vi "Cluster to String array.vi"(11 "input cluster":T11) -> (3 "appended array":string[][](array[string]))   [LabVIEW 2019, in "HardwareSetup_model001.lvlib" / "HardwareSetup_model001.lvclass"]
uses:
  HardwareSetup_model001.lvclass
  LIN.ctl
  Digital IO.ctl
  DMM.ctl
  Oscilloscope.ctl
  PLC.ctl
  ElectronicLoad.ctl
  PowerSupply.ctl
  CAN.ctl
  Programming.ctl
  Scanner.ctl
  HardwareSetup_model001.lvlib
panel:
  # "LIN_4"
  # "LIN_3"
  # "LIN_2"
  # "LIN_1"
  # "Digital IO_4"
  # "Digital IO_3"
  # "Digital IO_2"
  # "Digital IO_1"
  # "DMM_4"
  # "DMM_3"
  # "DMM_2"
  # "DMM_1"
  # "Oscilloscope_4"
  # "Oscilloscope_3"
  # "Oscilloscope_2"
  # "Oscilloscope_1"
  # "PLC_1"
  # "ElectronicLoad_4"
  # "ElectronicLoad_3"
  # "ElectronicLoad_2"
  # "ElectronicLoad_1"
  # "PowerSupply_4"
  # "PowerSupply_3"
  # "PowerSupply_2"
  # "PowerSupply_1"
  # "CAN_4"
  # "CAN_3"
  # "CAN_2"
  # "CAN_1"
  # "Programming_2"
  # "Programming_1"
  # "Scanner_4"
  # "Scanner_3"
  # "Scanner_2"
  # "Scanner_1"
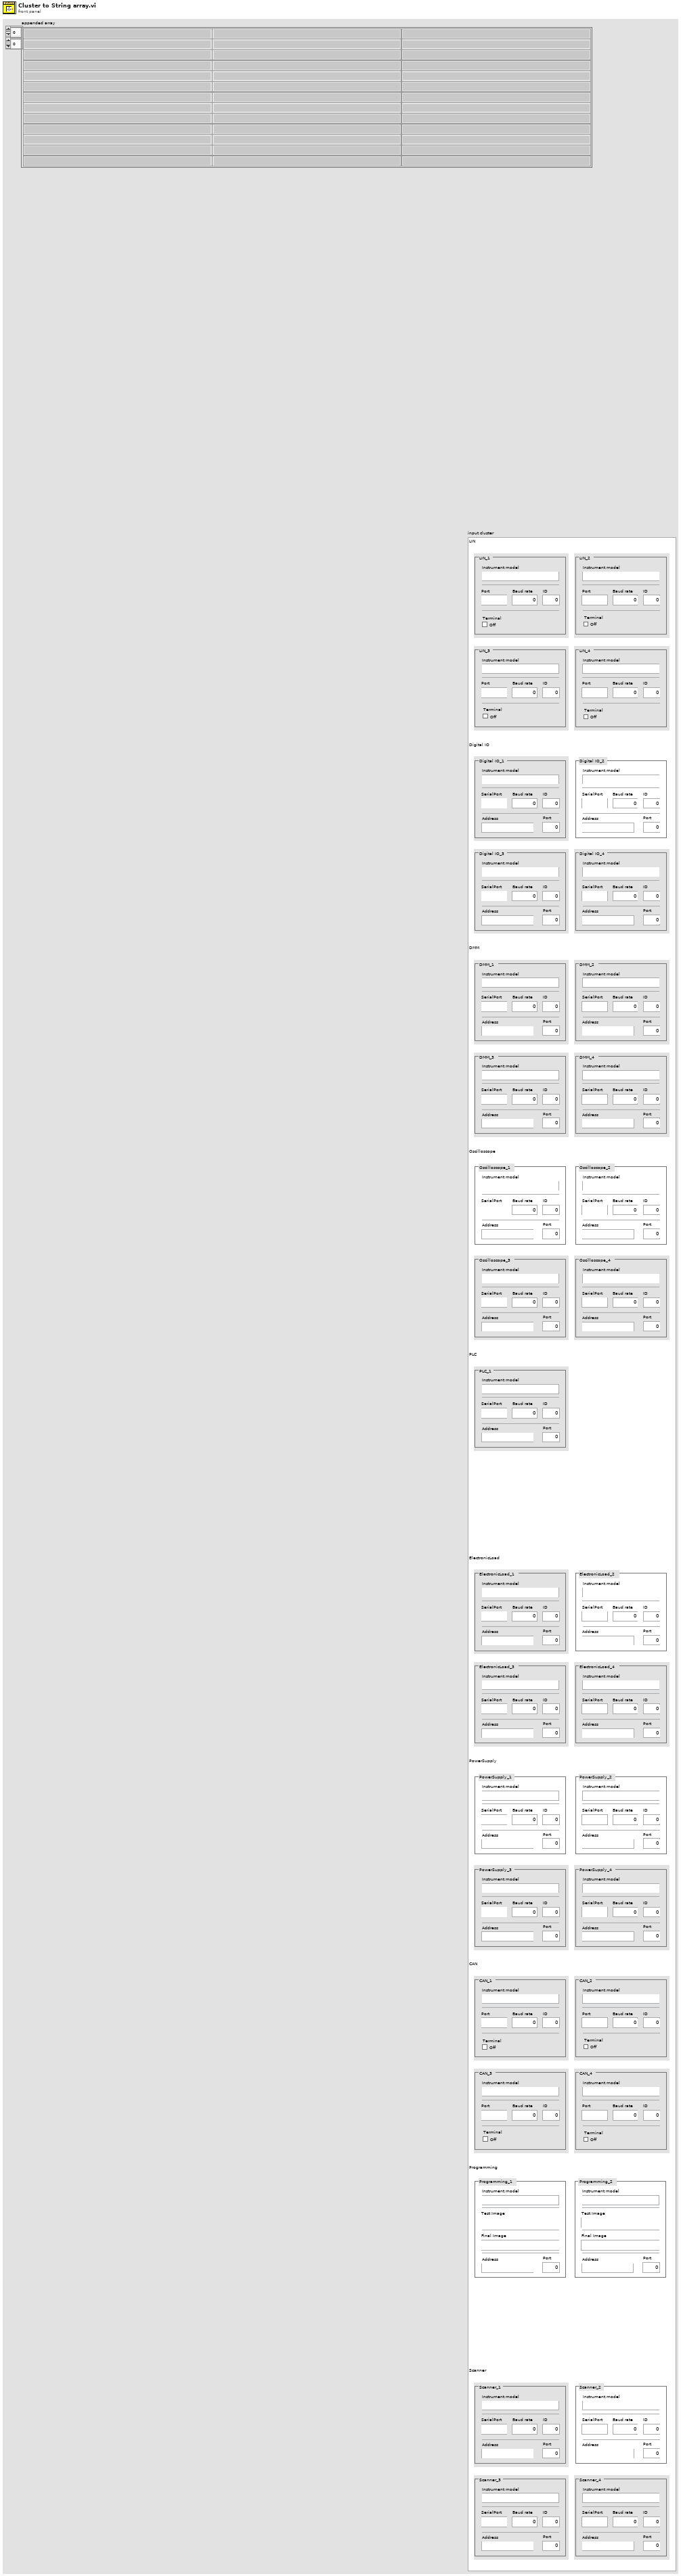
[diagram p1: front panel]
types:
  T1 = typedef "HardwareSetup_model001.lvlib/LIN.ctl" = cluster{"LIN 1":cluster{"Instrument model":string, "Port":string, "Baud rate":i32, "ID":i32, "Terminal":bool}, "LIN 2":cluster{"Instrument model":string, "Port":string, "Baud rate":i32, "ID":i32, "Terminal":bool}, "LIN 3":cluster{"Instrument model":string, "Port":string, "Baud rate":i32, "ID":i32, "Terminal":bool}, "LIN 4":cluster{"Instrument model":string, "Port":string, "Baud rate":i32, "ID":i32, "Terminal":bool}}
  T2 = typedef "HardwareSetup_model001.lvlib/Digital IO.ctl" = cluster{"Digital IO 1":cluster{"SerialPort":string, "Baud rate":i32, "Address":string, "ID":i32, "Port":i32, "Instrument model":string}, "Digital IO 2":cluster{"SerialPort":string, "Baud rate":i32, "Address":string, "ID":i32, "Port":i32, "Instrument model":string}, "Digital IO 3":cluster{"SerialPort":string, "Baud rate":i32, "Address":string, "ID":i32, "Port":i32, "Instrument model":string}, "Digital IO 4":cluster{"SerialPort":string, "Baud rate":i32, "Address":string, "ID":i32, "Port":i32, "Instrument model":string}}
  T3 = typedef "HardwareSetup_model001.lvlib/DMM.ctl" = cluster{"DMM 1":cluster{"SerialPort":string, "Baud rate":i32, "Address":string, "ID":i32, "Port":i32, "Instrument model":string}, "DMM 2":cluster{"SerialPort":string, "Baud rate":i32, "Address":string, "ID":i32, "Port":i32, "Instrument model":string}, "DMM 3":cluster{"SerialPort":string, "Baud rate":i32, "Address":string, "ID":i32, "Port":i32, "Instrument model":string}, "DMM 4":cluster{"SerialPort":string, "Baud rate":i32, "Address":string, "ID":i32, "Port":i32, "Instrument model":string}}
  T4 = typedef "HardwareSetup_model001.lvlib/Oscilloscope.ctl" = cluster{"Oscilloscope 1":cluster{"SerialPort":string, "Baud rate":i32, "Address":string, "ID":i32, "Port":i32, "Instrument model":string}, "Oscilloscope 2":cluster{"SerialPort":string, "Baud rate":i32, "Address":string, "ID":i32, "Port":i32, "Instrument model":string}, "Oscilloscope 3":cluster{"SerialPort":string, "Baud rate":i32, "Address":string, "ID":i32, "Port":i32, "Instrument model":string}, "Oscilloscope 4":cluster{"SerialPort":string, "Baud rate":i32, "Address":string, "ID":i32, "Port":i32, "Instrument model":string}}
  T5 = typedef "HardwareSetup_model001.lvlib/PLC.ctl" = cluster{"PLC 1":cluster{"SerialPort":string, "Baud rate":i32, "Address":string, "ID":i32, "Port":i32, "Instrument model":string}}
  T6 = typedef "HardwareSetup_model001.lvlib/ElectronicLoad.ctl" = cluster{"ElectronicLoad 1":cluster{"SerialPort":string, "Baud rate":i32, "Address":string, "ID":i32, "Port":i32, "Instrument model":string}, "ElectronicLoad 2":cluster{"SerialPort":string, "Baud rate":i32, "Address":string, "ID":i32, "Port":i32, "Instrument model":string}, "ElectronicLoad 3":cluster{"SerialPort":string, "Baud rate":i32, "Address":string, "ID":i32, "Port":i32, "Instrument model":string}, "ElectronicLoad 4":cluster{"SerialPort":string, "Baud rate":i32, "Address":string, "ID":i32, "Port":i32, "Instrument model":string}}
  T7 = typedef "HardwareSetup_model001.lvlib/PowerSupply.ctl" = cluster{"PowerSupply 1":cluster{"SerialPort":string, "Baud rate":i32, "Address":string, "ID":i32, "Port":i32, "Instrument model":string}, "PowerSupply 2":cluster{"SerialPort":string, "Baud rate":i32, "Address":string, "ID":i32, "Port":i32, "Instrument model":string}, "PowerSupply 3":cluster{"SerialPort":string, "Baud rate":i32, "Address":string, "ID":i32, "Port":i32, "Instrument model":string}, "PowerSupply 4":cluster{"SerialPort":string, "Baud rate":i32, "Address":string, "ID":i32, "Port":i32, "Instrument model":string}}
  T8 = typedef "HardwareSetup_model001.lvlib/CAN.ctl" = cluster{"CAN 1":cluster{"Instrument model":string, "Port":string, "Baud rate":i32, "ID":i32, "Terminal":bool}, "CAN 2":cluster{"Instrument model":string, "Port":string, "Baud rate":i32, "ID":i32, "Terminal":bool}, "CAN 3":cluster{"Instrument model":string, "Port":string, "Baud rate":i32, "ID":i32, "Terminal":bool}, "CAN 4":cluster{"Instrument model":string, "Port":string, "Baud rate":i32, "ID":i32, "Terminal":bool}}
  T9 = typedef "HardwareSetup_model001.lvlib/Programming.ctl" = cluster{"Programming 1":cluster{"Test Image":string, "Address":string, "Port":i32, "Instrument model":string, "Final Image":string}, "Programming 2":cluster{"Test Image":string, "Address":string, "Port":i32, "Instrument model":string, "Final Image":string}}
  T10 = typedef "HardwareSetup_model001.lvlib/Scanner.ctl" = cluster{"Scanner 1":cluster{"SerialPort":string, "Baud rate":i32, "Address":string, "ID":i32, "Port":i32, "Instrument model":string}, "Scanner 2":cluster{"SerialPort":string, "Baud rate":i32, "Address":string, "ID":i32, "Port":i32, "Instrument model":string}, "Scanner 3":cluster{"SerialPort":string, "Baud rate":i32, "Address":string, "ID":i32, "Port":i32, "Instrument model":string}, "Scanner 4":cluster{"SerialPort":string, "Baud rate":i32, "Address":string, "ID":i32, "Port":i32, "Instrument model":string}}
  T11 = cluster{"LIN":T1, "Digital IO":T2, "DMM":T3, "Oscilloscope":T4, "PLC":T5, "ElectronicLoad":T6, "PowerSupply":T7, "CAN":T8, "Programming":T9, "Scanner":T10}
  T12 = cluster{"SerialPort":string, "Baud rate":i32, "Address":string, "ID":i32, "Port":i32, "Instrument model":string}[]
  T13 = cluster{"Instrument model":string, "Port":string, "Baud rate":i32, "ID":i32, "Terminal":bool}[]
  T14 = cluster{"Test Image":string, "Address":string, "Port":i32, "Instrument model":string, "Final Image":string}[]
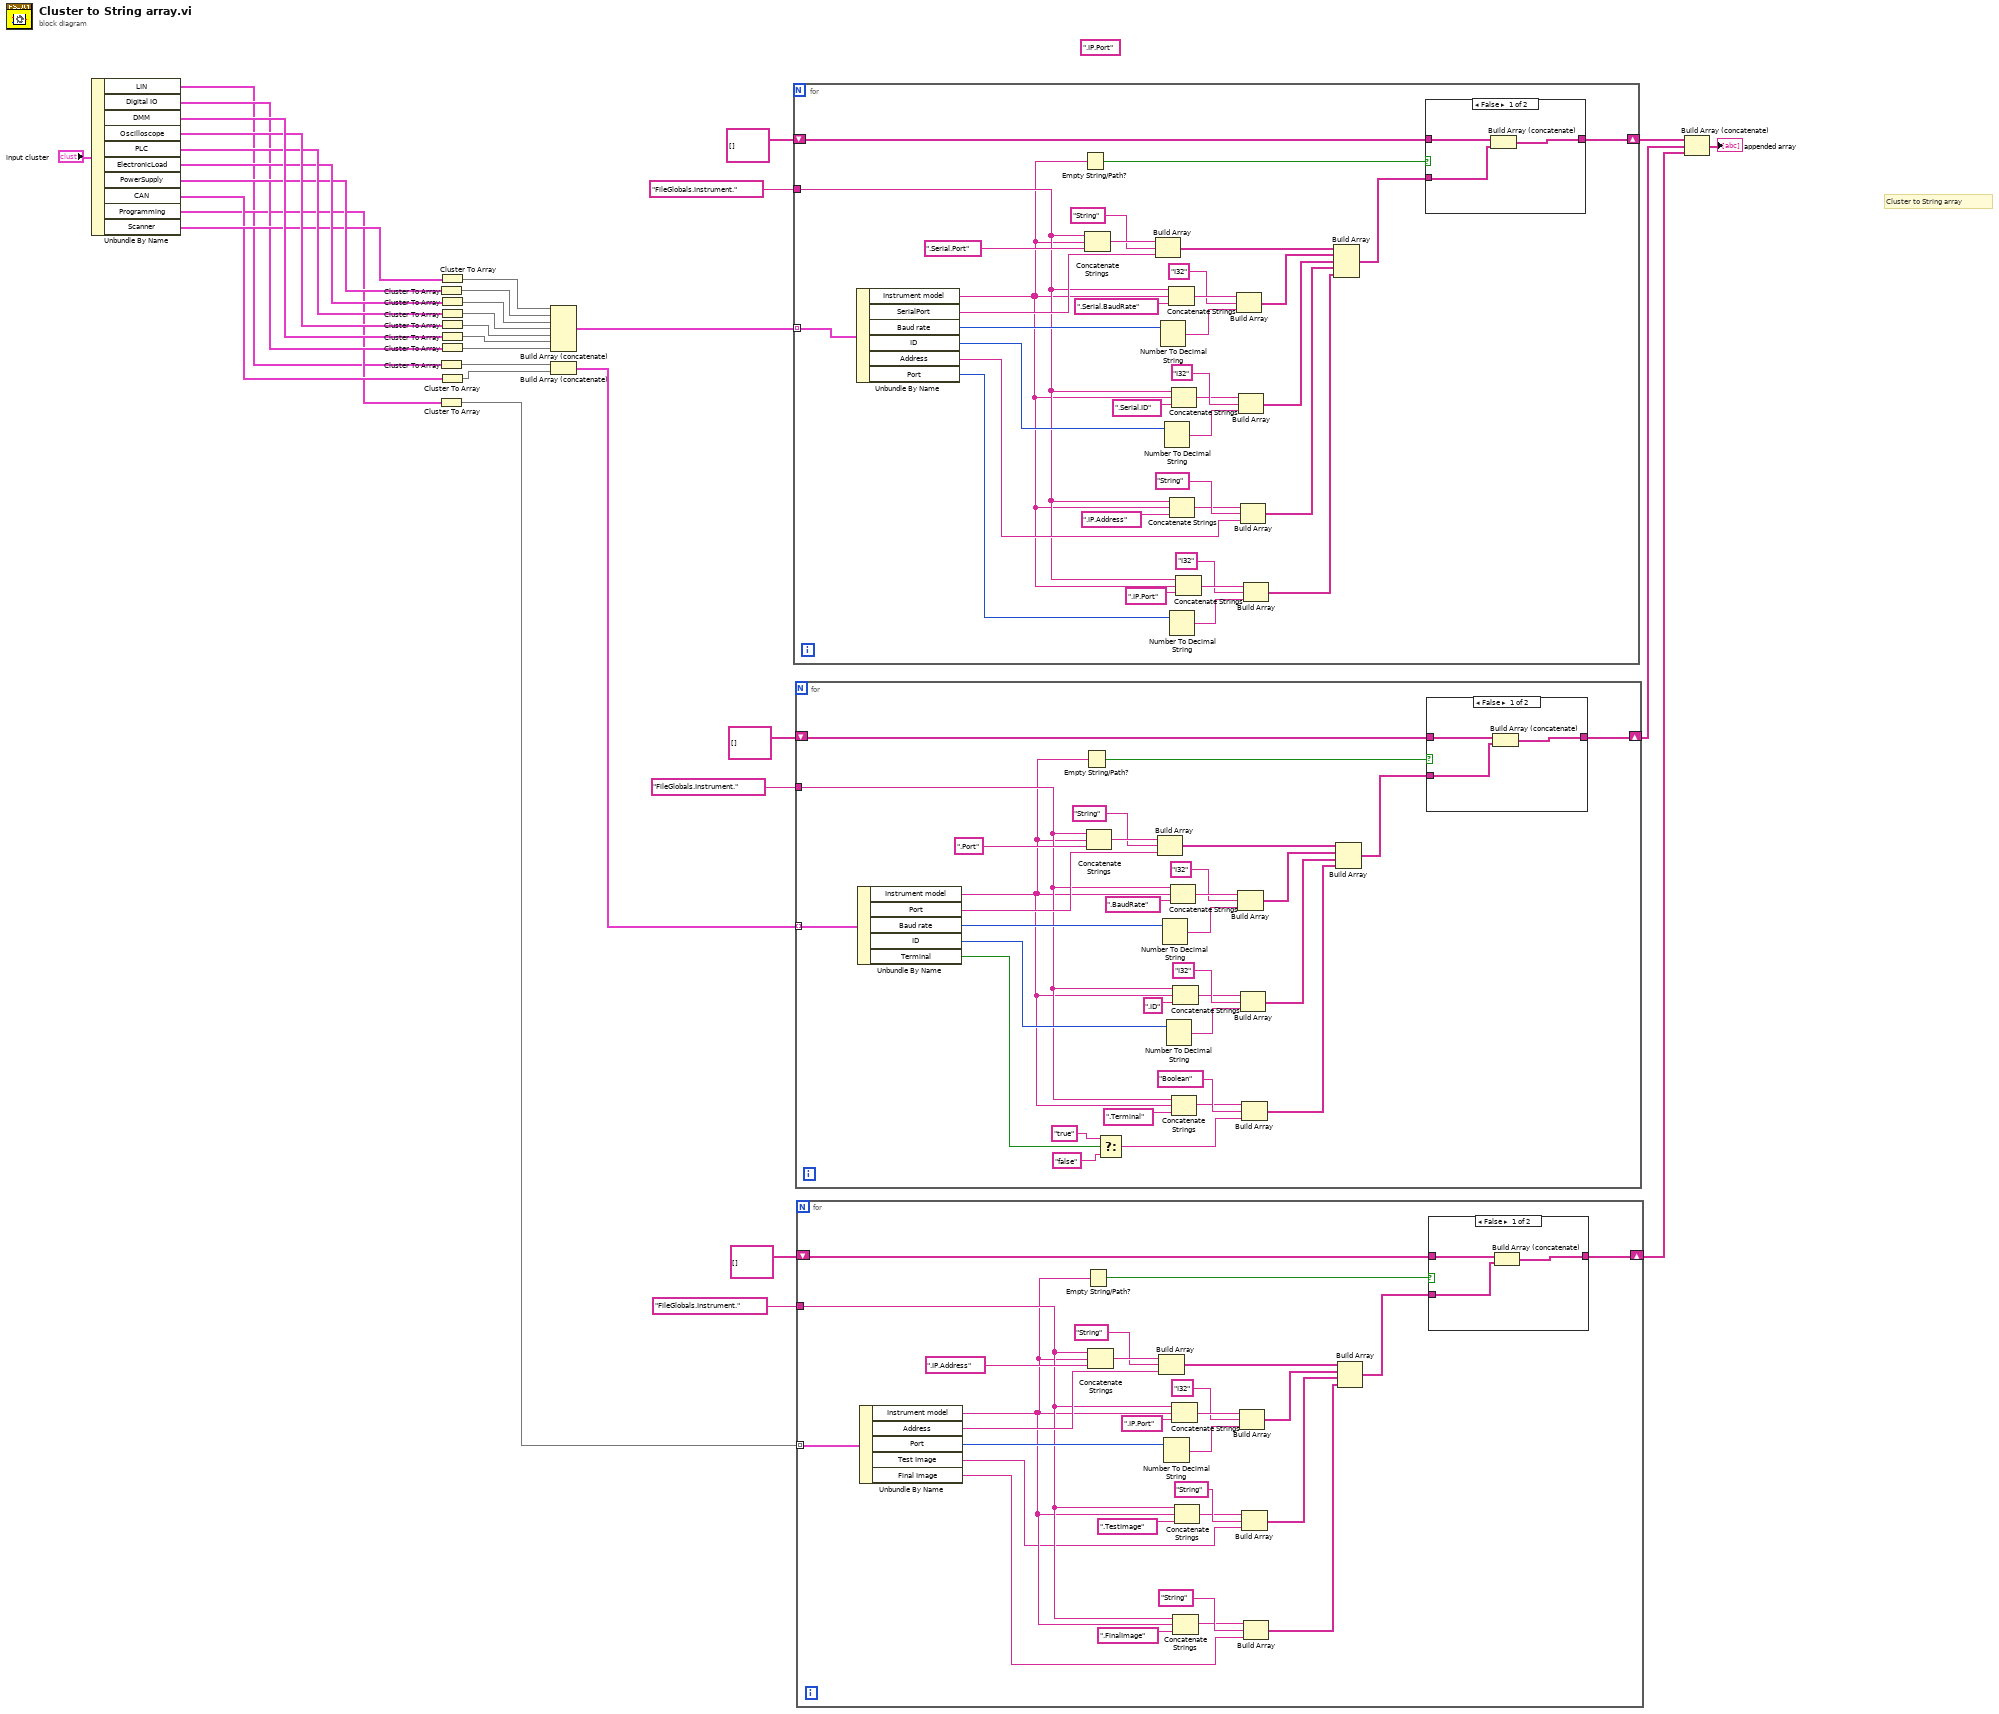
[diagram p0: block diagram]
diagram:
  (unwired) ".IP.Port" ("Lookup String")
  # "Cluster to String array"
  n1 = Unbundle By Name("input cluster") -> ("LIN"=w4:T1, "Digital IO"=w20:T2, "DMM"=w33:T3, "Oscilloscope"=w30:T4, "PLC"=w28:T5, "ElectronicLoad"=w26:T6, "PowerSupply"=w24:T7, "CAN"=w19:T8, "Programming"=w10:T9, "Scanner"=w22:T10)
  n2 = Cluster To Array(cluster=w24) -> (array=w23:T12)
  n3 = Cluster To Array(cluster=w4) -> (array=w18:T13)
  n4 = Cluster To Array(cluster=w10) -> (array=w5:T14)
  n5 = Cluster To Array(cluster=w22) -> (array=w21:T12)
  n6 = Cluster To Array(cluster=w26) -> (array=w25:T12)
  n7 = Cluster To Array(cluster=w28) -> (array=w27:T12)
  n8 = Cluster To Array(cluster=w30) -> (array=w29:T12)
  n9 = Cluster To Array(cluster=w33) -> (array=w31:T12)
  n10 = Cluster To Array(cluster=w20) -> (array=w32:T12)
  n11 = Cluster To Array(cluster=w19) -> (array=w17:T13)
  n12 = Build Array (concatenate)(w21, w23, w25, w27, w29, w31, w32) -> (w16:T12)
  n13 = Build Array (concatenate)(w18, w17) -> (w11:T13)
  n14 = for {
    tunnel: w16 -> [w68] mode=indexing
    tunnel: "FileGlobals.Instrument." ("Lookup String") -> [w42]
    shift-right: [w35] -> w9
    shift-left: string[][] [] -> [w37]
    n15 = Unbundle By Name(w68) -> ("Instrument model"=w41:string, "SerialPort"=w64:string, "Baud rate"=w60:i32, "ID"=w52:i32, "Address"=w47:string, "Port"=w39:i32)
    n16 = Empty String/Path?(string/path=w41) -> (empty?=w38:bool)
    n17 = Concatenate Strings(w42, w41, ".Serial.Port" ("Lookup String")) -> (w66:string)
    n18 = Build Array(w66, "String", w64) -> (w58:string[])
    n19 = Number To Decimal String(number=w60) -> (decimal integer string=w59:string)  [unwired: 1 in]
    n20 = Number To Decimal String(number=w52) -> (decimal integer string=w56:string)  [unwired: 1 in]
    n21 = Concatenate Strings(w42, w41, ".Serial.BaudRate" ("Lookup String")) -> (w62:string)
    n22 = Concatenate Strings(w42, w41, ".IP.Address" ("Lookup String")) -> (w49:string)
    n23 = Number To Decimal String(number=w39) -> (decimal integer string=w40:string)  [unwired: 1 in]
    n24 = Concatenate Strings(w42, w41, ".Serial.ID" ("Lookup String")) -> (w54:string)
    n25 = Concatenate Strings(w42, w41, ".IP.Port" ("Lookup String")) -> (w44:string)
    n26 = Build Array(w62, "I32", w59) -> (w57:string[])
    n27 = Build Array(w54, "I32", w56) -> (w51:string[])
    n28 = Build Array(w49, "String", w47) -> (w46:string[])
    n29 = Build Array(w44, "I32", w40) -> (w34:string[])
    n30 = Build Array(w58, w57, w51, w46, w34) -> (w36:string[][])
    n31 = case shown="False" w38 {
      tunnel: w37 -> [w71 w72]
      tunnel: w36 -> [w70 _]
      tunnel: [w69 w72] -> w35
      frame False {
        n32 = Build Array (concatenate)(w71, w70) -> (w69:string[][])
      }
      frame True {
      }
    }
  }
  n33 = for {
    tunnel: w11 -> [w104] mode=indexing
    tunnel: "FileGlobals.Instrument." ("Lookup String") -> [w82]
    shift-right: [w77] -> w8
    shift-left: string[][] [] -> [w79]
    n34 = Unbundle By Name(w104) -> ("Instrument model"=w81:string, "Port"=w100:string, "Baud rate"=w96:i32, "ID"=w88:i32, "Terminal"=w76:bool)
    n35 = Empty String/Path?(string/path=w81) -> (empty?=w80:bool)
    n36 = Concatenate Strings(w82, w81, ".Port" ("Lookup String")) -> (w102:string)
    n37 = Select(t="true", s=w76, f="false") -> (s? t:f=w73:string)
    n38 = Build Array(w102, "String", w100) -> (w94:string[])
    n39 = Number To Decimal String(number=w96) -> (decimal integer string=w95:string)  [unwired: 1 in]
    n40 = Number To Decimal String(number=w88) -> (decimal integer string=w92:string)  [unwired: 1 in]
    n41 = Concatenate Strings(w82, w81, ".BaudRate" ("Lookup String")) -> (w98:string)
    n42 = Concatenate Strings(w82, w81, ".Terminal" ("Lookup String")) -> (w85:string)
    n43 = Concatenate Strings(w82, w81, ".ID" ("Lookup String")) -> (w90:string)
    n44 = Build Array(w98, "I32", w95) -> (w93:string[])
    n45 = Build Array(w90, "I32", w92) -> (w87:string[])
    n46 = Build Array(w85, "Boolean", w73) -> (w83:string[])
    n47 = Build Array(w94, w93, w87, w83) -> (w78:string[][])
    n48 = case shown="False" w80 {
      tunnel: w79 -> [w107 w108]
      tunnel: w78 -> [w106 _]
      tunnel: [w105 w108] -> w77
      frame False {
        n49 = Build Array (concatenate)(w107, w106) -> (w105:string[][])
      }
      frame True {
      }
    }
  }
  n50 = for {
    tunnel: w5 -> [w136] mode=indexing
    tunnel: "FileGlobals.Instrument." ("Lookup String") -> [w116]
    shift-right: [w111] -> w3
    shift-left: string[][] [] -> [w113]
    n51 = Unbundle By Name(w136) -> ("Instrument model"=w115:string, "Address"=w132:string, "Port"=w128:i32, "Test Image"=w110:string, "Final Image"=w109:string)
    n52 = Empty String/Path?(string/path=w115) -> (empty?=w114:bool)
    n53 = Concatenate Strings(w116, w115, ".IP.Address" ("Lookup String")) -> (w134:string)
    n54 = Build Array(w134, "String", w132) -> (w126:string[])
    n55 = Number To Decimal String(number=w128) -> (decimal integer string=w127:string)  [unwired: 1 in]
    n56 = Concatenate Strings(w116, w115, ".IP.Port" ("Lookup String")) -> (w130:string)
    n57 = Concatenate Strings(w116, w115, ".FinalImage" ("Lookup String")) -> (w119:string)
    n58 = Concatenate Strings(w116, w115, ".TestImage" ("Lookup String")) -> (w123:string)
    n59 = Build Array(w130, "I32", w127) -> (w125:string[])
    n60 = Build Array(w123, "String", w110) -> (w121:string[])
    n61 = Build Array(w119, "String", w109) -> (w117:string[])
    n62 = Build Array(w126, w125, w121, w117) -> (w112:string[][])
    n63 = case shown="False" w114 {
      tunnel: w113 -> [w139 w140]
      tunnel: w112 -> [w138 _]
      tunnel: [w137 w140] -> w111
      frame False {
        n64 = Build Array (concatenate)(w139, w138) -> (w137:string[][])
      }
      frame True {
      }
    }
  }
  n65 = Build Array (concatenate)(w9, w8, w3) -> (→"appended array":string[][])
